vi "PropertyNode.vi"() -> ()   [LabVIEW 2023]
panel:
  in  "Blank Button 2":bool
  in  "Blank Button":bool
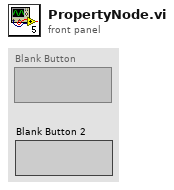
[diagram p1: front panel]
types:
  T1 = enum8{"Enabled", "Disabled", "Disabled and Grayed Out"}
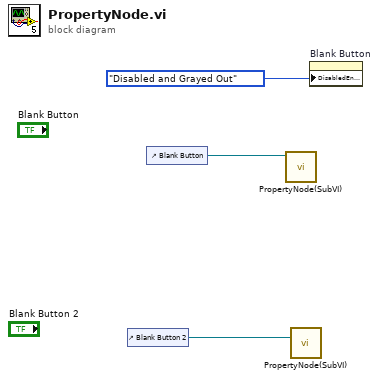
[diagram p0: block diagram]
diagram:
  n1 = control-ref of="Blank Button 2"() -> (w2:refnum<vi>)
  n2 = control-ref of="Blank Button"() -> (w3:refnum<vi>)
  n3 = call "PropertyNode(SubVI).vi"("Boolean in"=w3) -> ()  [unwired: 11 in]
  n4 = call "PropertyNode(SubVI).vi"("Boolean in"=w2) -> ()  [unwired: 11 in]
  n5 = property on="Blank Button" class="Bool"("DisabledEnum"=T1."Disabled and Grayed Out" ("Disabled")) -> ()  [unwired: 2 in, 2 out]
